vi "Read.vi"(7 "Enable Sound":bool, 8 "error in (no error)":errorcluster, 9 "Audio Channels":cluster{"Channel":i32}, 11 "Electrophysiology in":refnum<class "Electrophysiology.lvclass">) -> (0 "error out":errorcluster, 2 "Samples":u32, 3 "Electrophysiology out":refnum<class "Electrophysiology.lvclass">)   [LabVIEW 2010, in "Electrophysiology.lvclass"]
uses:
  Electrophysiology.lvclass
  Electrophysiology.lvclass/Electrophysiology.ctl
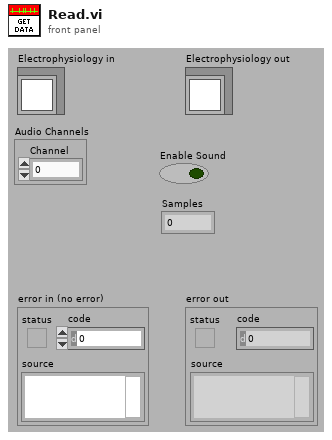
[diagram p1: front panel]
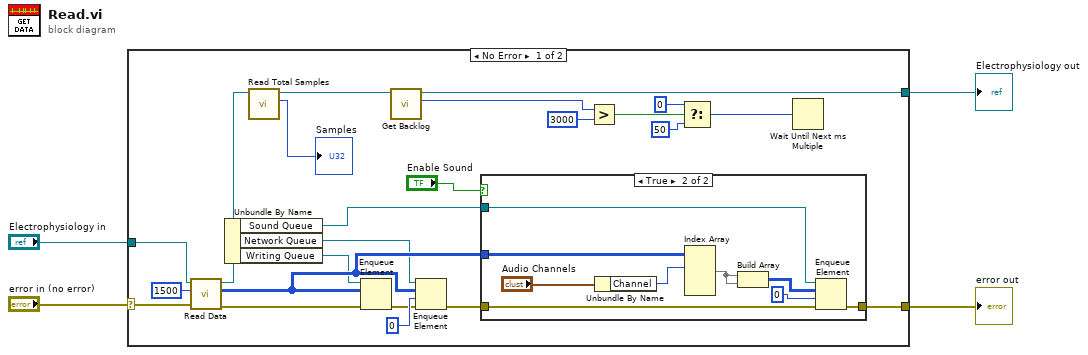
[diagram p0: block diagram]
diagram:
  n1 = case shown="No Error" "error in (no error)" {
    selector: "error in (no error)" -> [w25 w39]
    tunnel: [w27 w39] -> w3
    tunnel: [w6 w38] -> w1
    tunnel: "Electrophysiology in" -> [w26 w38]
    frame No Error {
      n2 = call-dynamic "Read Data.vi"("error in (no error)"=w25, "Read Size"=1500, "AcquireTraces in"=w26) -> ("error out"=w24:errorcluster, "data"=w21:i32[][], "AcquireTraces out"=w23:refnum<class "Electrophysiology.lvclass">)  [unwired: 6 in]
      n3 = Unbundle By Name(w23) -> ("Sound Queue"=w15:refnum<queue>, "Network Queue"=w19:refnum<queue>, "Writing Queue"=w18:refnum<queue>)
      n4 = call-dynamic "Read Total Samples.vi"("AcquireTraces in"=w23) -> ("Total Samples"=→"Samples":u64, "AcquireTraces out"=w7:refnum<class "Electrophysiology.lvclass">)  [unwired: 8 in, 1 out]
      n5 = Enqueue Element(queue=w18, element=w21, error in (no error)=w24) -> (error out=w17:errorcluster)  [unwired: 1 in, 2 out]
      n6 = call-dynamic "Get Backlog.vi"("AcquireTraces in"=w7) -> ("Backlog"=w5:u32, "AcquireTraces out"=w6:refnum<class "Electrophysiology.lvclass">)  [unwired: 8 in, 1 out]
      n7 = Enqueue Element(queue=w19, element=w21, timeout in ms (-1)=0, error in (no error)=w17) -> (error out=w16:errorcluster)  [unwired: 2 out]
      n8 = case shown="True" "Enable Sound" {
        tunnel: w15 -> [_ w35]
        tunnel: w16 -> [w28 w34]
        tunnel: [w28 w32] -> w27
        tunnel: w21 -> [_ w31]
        frame False {
        }
        frame True {
          n9 = Unbundle By Name("Audio Channels") -> ("Channel"=w37:i32)
          n10 = Index Array(array=w31, index (row) #1=w37) -> (element #1=w29:i32[])  [unwired: 3 in, 1 out]
          n11 = Build Array(w29, w29) -> (w30:i32[][])
          n12 = Enqueue Element(queue=w35, element=w30, timeout in ms (-1)=0, error in (no error)=w34) -> (error out=w32:errorcluster)  [unwired: 2 out]
        }
      }
      n13 = Greater?(x=w5, y=u32 3000) -> (0:w11:bool)
      n14 = Select(t=0, s=w11, f=u32 50 ("millisecond multiple")) -> (s? t:f=w8:u32)
      n15 = Wait Until Next ms Multiple(millisecond multiple=w8) -> ()  [unwired: 1 out]
    }
    frame Error {
    }
  }
  "error out" <- w3
  "Electrophysiology out" <- w1
